vi "Services.Compile.Comm.State.GetDefault.vi"(8 "error in (no error)":errorcluster, 11 "Section Ref in":T1 format="%.0x") -> (0 "error out":errorcluster, 2 "Initial Comm State":bool, 3 "Section Ref out":T1 format="%.0x")   [LabVIEW 2019, in "Diagnostics Addon System Explorer.lvlib"]
uses:
  Diagnostics Addon System Explorer.lvlib
  <vilib>/NI VeriStand/Custom Device Tools/Custom Device Utility Library/Custom Device Utility Library.lvlib
  Addon Shared/Types/Type.ctl
  Addon Shared/Diagnostics Addon Shared.lvlib
  <vilib>/NI VeriStand/Custom Device Tools/Custom Device Utility Library/NI VeriStand - Search for Item by GUID.vi
  <vilib>/NI VeriStand/Custom Device API/Custom Device API.lvlib
  <vilib>/NI VeriStand/Custom Device API/Custom Device Item Ref.ctl
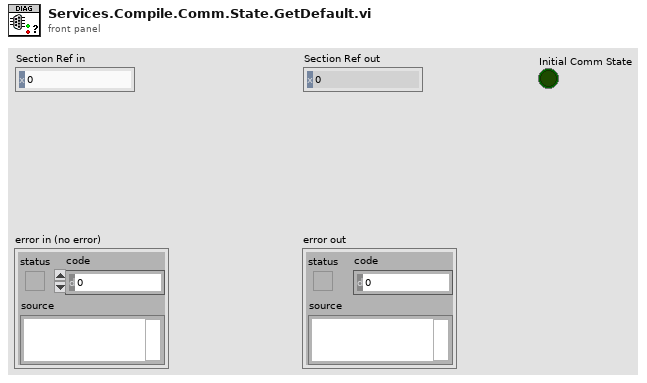
[diagram p1: front panel]
types:
  T1 = typedef "Custom Device API.lvlib/Custom Device Item Ref.ctl" = u64
  T2 = typedef "Diagnostics Addon Shared.lvlib/Type.ctl" = enum16{"DID", "CDID", "PID", "CPID", "Read Memory", "Write Memory", "IO Control", "Routine Start", "Routine Request", "Routine Stop", "User Defined", "DTC Control", "Clear DTCs", "Read DTCs", "Start DTCs", "DTC Change Count", "Tester Present", "Unlock ECU", "Reset ECU", "Diag Session Control", "Communication Control", "DPID Control", "Poll Control", "Diag Comm Port Control"}
  T3 = typedef "Custom Device API.lvlib/Custom Device Channel.ctl" = cluster{"Type":T4, "Units":string, "Default Value":dbl, "Faultable":bool, "Scalable":bool}
  T4 = typedef "Custom Device API.lvlib/Custom Device Channel Type.ctl" = enum16{"Input", "Output"}
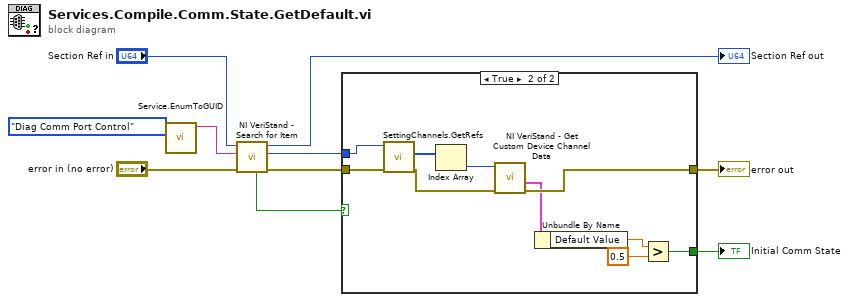
[diagram p0: block diagram]
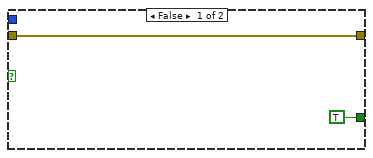
[diagram p2: hidden frame]
diagram:
  n1 = call "Service.EnumToGUID.vi"("Type"=Type."Diag Comm Port Control") -> ("GUID"=w3:string)  [unwired: 10 in]
  n2 = call-poly <vilib>:"NI VeriStand - Search for Item.vi"("error in"="error in (no error)", "Item GUID"=w3, "Section Ref in"="Section Ref in") -> ("error out"=w5:errorcluster, "Item Ref"=w6:T1, "Section Ref out"=→"Section Ref out":T1, "Found"=w4:bool)  [unwired: 5 in]
  n3 = case shown="True" w4 {
    tunnel: [w12 w17] -> w9
    tunnel: w6 -> [_ w21]
    tunnel: w5 -> [w12 w22]
    tunnel: [TRUE w13] -> w1
    frame False {
    }
    frame True {
      n4 = call "SettingChannels.GetRefs.vi"("error in (no error)"=w22, "Item Ref in"=w21) -> ("error out"=w18:errorcluster, "Settings"=w20:T1[])  [unwired: 7 in, 1 out]
      n5 = Index Array(array=w20) -> (element=w19:T1)  [unwired: 1 in]
      n6 = call <vilib>:"NI VeriStand - Get Custom Device Channel Data.vi"("error in (no error)"=w18, "Channel Ref in"=w19) -> ("error out"=w17:errorcluster, "Channel"=w16:T3)  [unwired: 4 in, 4 out]
      n7 = Unbundle By Name(w16) -> ("Default Value"=w15:dbl)
      n8 = Greater?(x=w15, y=0.5) -> (0:w13:bool)
    }
  }
  "error out" <- w9
  "Initial Comm State" <- w1
